vi "Main.Constants.vi"() -> ()   [LabVIEW 2013, in "Simple Sequence Tools - Shared.lvlib"]
uses:
  Simple Sequence Tools - Shared.lvlib
  <vilib>/Utility/miscctls.llb/LVBoundsTypeDef.ctl
  Types/Sequence.Reference.ctl
panel:
  in  "INI.FileName":string="Settings.INI"
  in  "Task.StepManagePrefix":string="StepManage_"
  in  "Task.StepExePrefix":string="StepExe_"
  in  "Sequence.ForLoopBaseVar":string="i"
  in  "Task.Abort":string="Abort"
  in  "Task.Sequence":string="Sequence"
  in  "Sequence.TempStepInfo":string="TempStepInfo"
  in  "Sequence.StartingStep":string="SequenceStartingStep"
  in  "Sequence.StartingIteration":string="SequenceStartingIteration"
  in  "References":T1[](array[typedef])=[{"Name"="Ramp", "RelativePath"="\\nivs.lib\\Sequence Library\\Standard\\Waveforms\\Ramp.nivsseq"}, {"Name"="Wait", "RelativePath"="\\nivs.lib\\Sequence Library\\Standard\\Timing\\Wait.nivsseq"}]
  in  "Sequence.NewChannelSize":T2={"Width"=175, "Height"=0}
  in  "Sequence.BaseHeaderSize":T2[](array[typedef])=[{"Width"=81, "Height"=0}, {"Width"=56, "Height"=0}, {"Width"=300, "Height"=0}, {"Width"=2500, "Height"=0}]
  in  "Sequence.BaseHeader":string[](array[string])=["Step\nDuration (secs)", "Operator", "Additional Condition(s)"]
  in  "iStep.Syntax":string="iStep (StartVal, EndVal, StepVal)"
  in  "Menu.PropertyPrefix":string="Property."
  in  "Menu.ConditionsPrefix":string="Conditions."
  in  "NoChange.Syntax":string="Unchanged"
  in  "Menu.StepPrefix":string="Step."
  in  "Ramp.Syntax":string="Ramp (StartVal, EndVal)"
  in  "Step.Syntax":string="Step (Val)"
  in  "# of Static Columns":u32=3
  in  "Menu.ChannelPrefix":string="Channel."
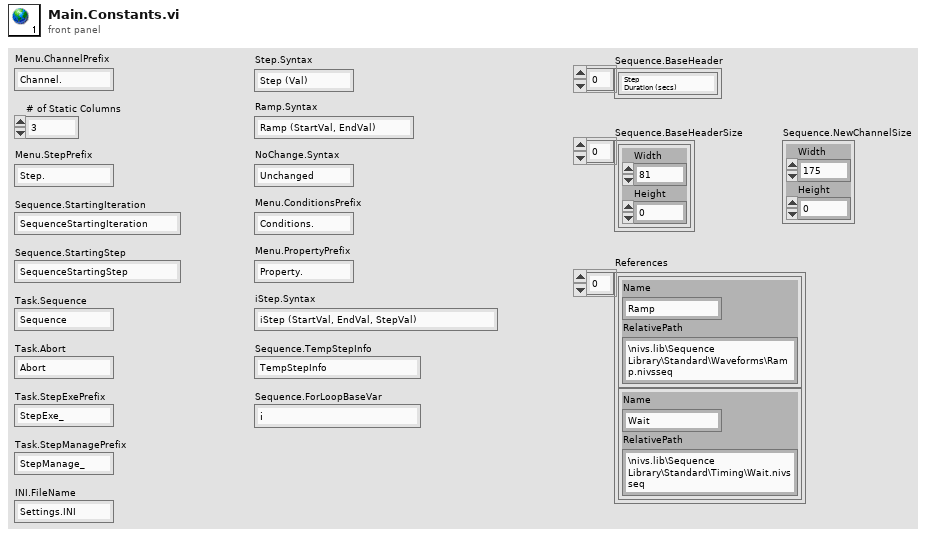
[diagram p1: front panel]
types:
  T1 = typedef "Simple Sequence Tools - Shared.lvlib/Sequence.Reference.ctl" = cluster{"Name":string, "RelativePath":string}
  T2 = typedef "LVBoundsTypeDef.ctl" = cluster{"Width":u32, "Height":u32}
diagram:
